vi "Registry FGV.vi"(7 "State (Get Logger)":T2(ring)=enum."Get Logger", 8 "error in (no error)":errorcluster, 9 "Debug Level in":T1, 10 "Sink":refnum<class "Sink.lvclass">, 11 "Name":string) -> (0 "error out":errorcluster, 1 "Debug Level out":T1, 2 "Sinks":refnum<class "Sink.lvclass">[](array[class]), 3 "Logger out":refnum<class "Logger.lvclass">)   [LabVIEW 2020, in "LV Logging.lvlib"]
uses:
  LV Logging.lvlib
  Logger/Logger.lvclass
  Sink/Sink.lvclass
  Registry/Registry.lvclass
  Type Defs/Debug Level.ctl
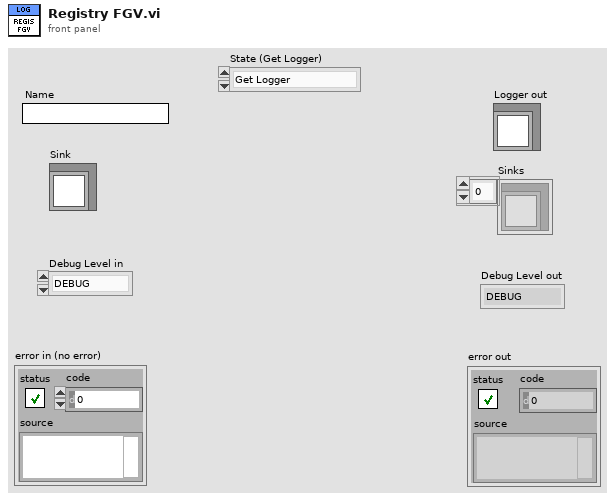
[diagram p1: front panel]
types:
  T1 = typedef "LV Logging.lvlib/Debug Level.ctl" = enum16{"DEBUG", "INFO", "WARN", "ERROR", "FATAL"}
  T2 = enum16{"Init", "Get Logger", "Register Sink", "Set Global Debug Level", "Get Sinks", "Get Global Debug Level"}
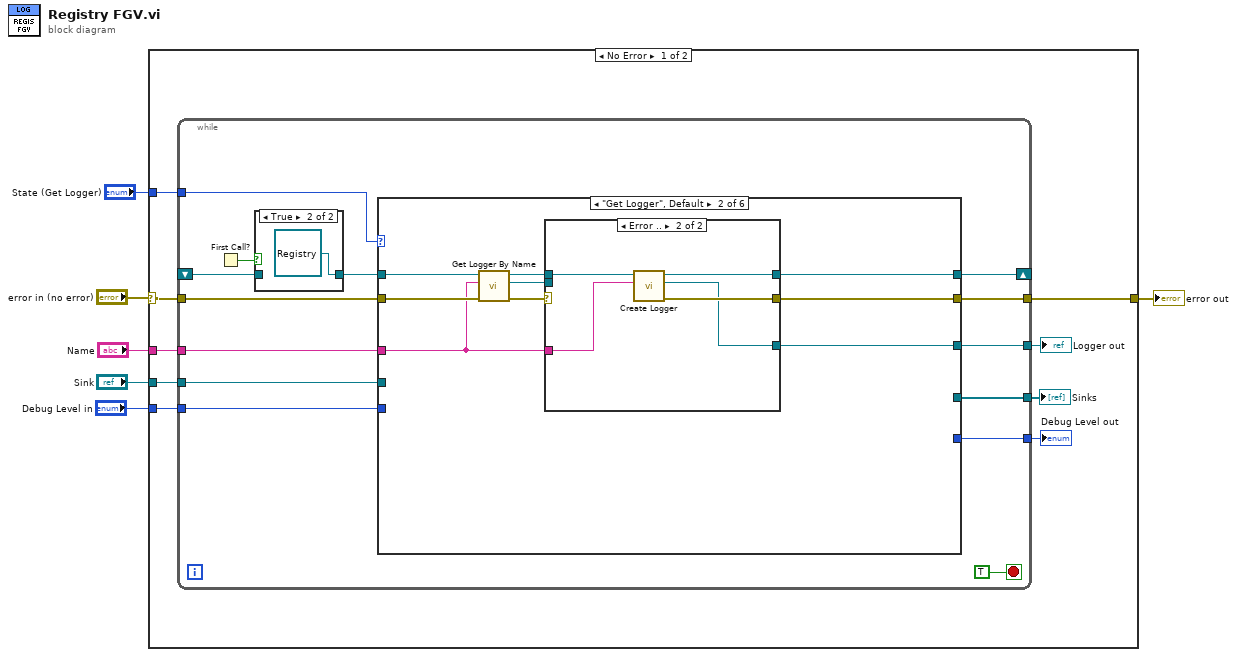
[diagram p0: block diagram]
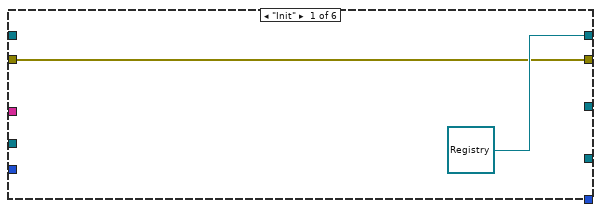
[diagram p3: hidden frame]
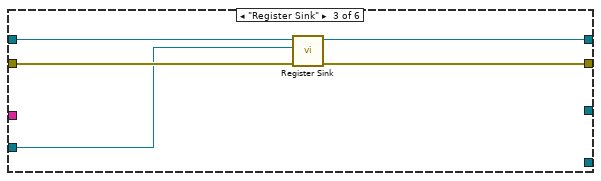
[diagram p5: hidden frame]
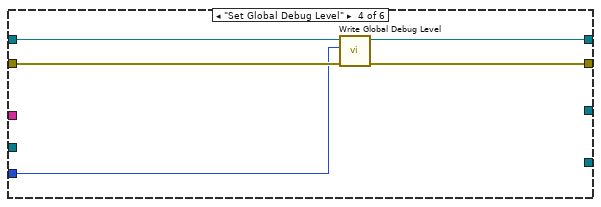
[diagram p6: hidden frame]
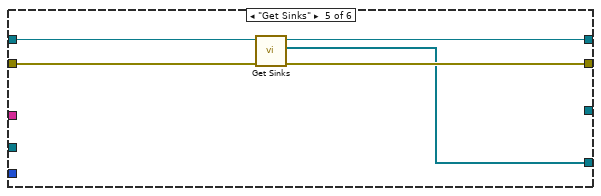
[diagram p7: hidden frame]
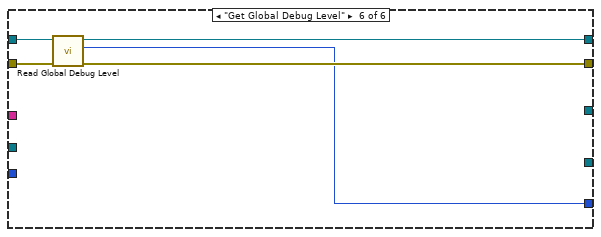
[diagram p8: hidden frame]
diagram:
  n1 = case shown="No Error" "error in (no error)" {
    selector: "error in (no error)" -> [w13 w71]
    tunnel: "State (Get Logger)" -> [w15 _]
    tunnel: "Name" -> [w14 _]
    tunnel: [w12 w71] -> w3
    tunnel: "Sink" -> [w10 _]
    tunnel: "Debug Level in" -> [w8 _]
    frame No Error {
      n2 = while {
        shift-right: [w28] -> _
        shift-left: _ -> [w20]
        tunnel: w15 -> [w27]
        tunnel: w14 -> [w26]
        tunnel: w13 -> [w25]
        tunnel: [w24] -> w12
        tunnel: [w23] -> w11
        tunnel: w10 -> [w22]
        tunnel: [w21] -> w9
        tunnel: w8 -> [w17]
        tunnel: [w16] -> w7
        stop <- TRUE stop-if-true
        n3 = First Call?() -> (First Call?: T/F=w18:bool)
        n4 = case shown="True" w18 {
          tunnel: w20 -> [w30 _]
          tunnel: [w30 refnum<class "Registry.lvclass"> refnum ("LV Logging.lvlib:Registry.lvclass")] -> w19
          frame False {
          }
          frame True {
          }
        }
        n5 = case shown="\"Get Logger\", Default" w27 {
          tunnel: [refnum<class "Registry.lvclass"> refnum ("LV Logging.lvlib:Registry.lvclass") w40 w53 w59 w62 w68] -> w28
          tunnel: w26 -> [_ w35 _ _ _ _]
          tunnel: w19 -> [_ w42 w54 w60 w64 w70]
          tunnel: w25 -> [w32 w37 w55 w58 w65 w69]
          tunnel: [w32 w36 w52 w57 w63 w67] -> w24
          tunnel: [_ w34 _ _ _ _] -> w23
          tunnel: w22 -> [_ _ w51 _ _ _]
          tunnel: [_ _ _ _ w61 _] -> w21
          tunnel: w17 -> [_ _ _ w56 _ _]
          tunnel: [_ _ _ _ _ w66] -> w16
          frame "Init" {
          }
          frame "Get Logger", Default {
            n6 = call "Get Logger By Name.vi"("error in (no error)"=w37, "Name"=w35, "Registry in"=w42) -> ("error out"=w39:errorcluster, "Logger"=w38:refnum<class "Logger.lvclass">, "Registry out"=w41:refnum<class "Registry.lvclass">)  [unwired: 6 in]
            n7 = case shown="Error .." w39 {
              selector: w39 -> [w44 _]
              tunnel: w41 -> [w45 w50]
              tunnel: [w45 w49] -> w40
              tunnel: w38 -> [w43 _]
              tunnel: [w44 w48] -> w36
              tunnel: w35 -> [_ w47]
              tunnel: [w43 w46] -> w34
              frame No Error {
              }
              frame Error {
                n8 = call "Create Logger.vi"("Name"=w47, "Registry in"=w50) -> ("error out"=w48:errorcluster, "Logger out"=w46:refnum<class "Logger.lvclass">, "Registry out"=w49:refnum<class "Registry.lvclass">)  [unwired: 7 in]
              }
            }
          }
          frame "Register Sink" {
            n9 = call "Register Sink.vi"("error in (no error)"=w55, "Sink"=w51, "Registry in"=w54) -> ("error out"=w52:errorcluster, "Registry out"=w53:refnum<class "Registry.lvclass">)  [unwired: 7 in]
          }
          frame "Set Global Debug Level" {
            n10 = call "Write Global Debug Level.vi"("error in (no error)"=w58, "Debug Level"=w56, "Registry in"=w60) -> ("error out"=w57:errorcluster, "Registry out"=w59:refnum<class "Registry.lvclass">)  [unwired: 7 in]
          }
          frame "Get Sinks" {
            n11 = call "Get Sinks.vi"("error in (no error)"=w65, "Registry in"=w64) -> ("error out"=w63:errorcluster, "Sinks"=w61:refnum<class "Sink.lvclass">[], "Registry out"=w62:refnum<class "Registry.lvclass">)  [unwired: 7 in]
          }
          frame "Get Global Debug Level" {
            n12 = call "Read Global Debug Level.vi"("error in (no error)"=w69, "Registry in"=w70) -> ("error out"=w67:errorcluster, "Debug Level"=w66:T1, "Registry out"=w68:refnum<class "Registry.lvclass">)  [unwired: 7 in]
          }
        }
      }
      "Logger out" <- w11
      "Sinks" <- w9
      "Debug Level out" <- w7
    }
    frame Error {
    }
  }
  "error out" <- w3
